vi "Set_Input_file.vi"() -> (2 "输出文件名称":string)   [LabVIEW 2018]
panel:
  in  "版本":string
  in  "输入文件名称：":string
  in  "停止":bool
  in  "确定":bool
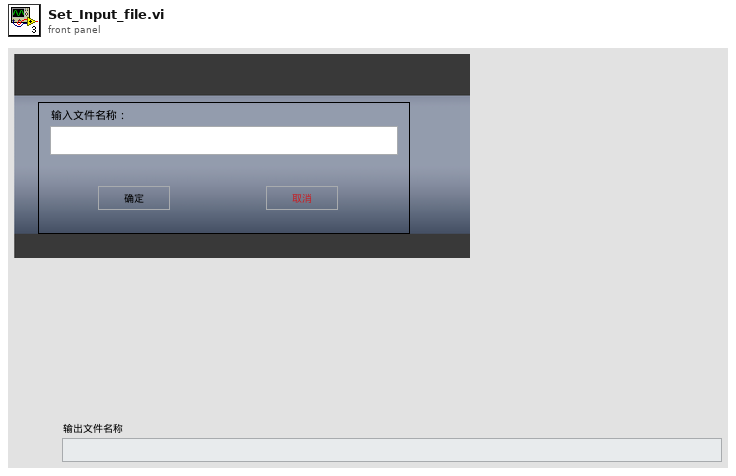
[diagram p1: front panel]
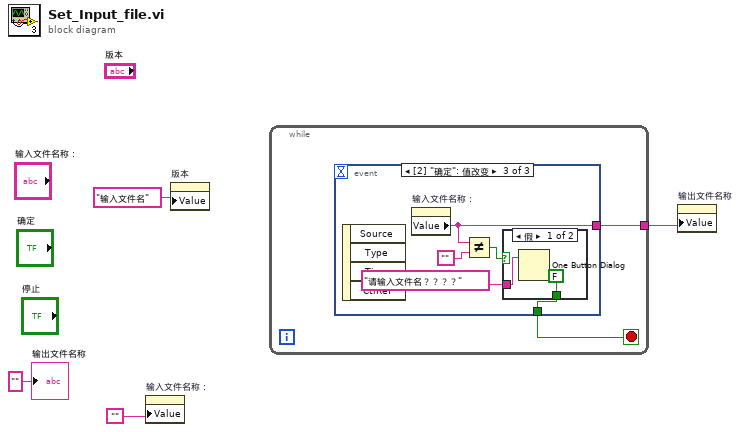
[diagram p0: block diagram]
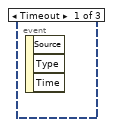
[diagram p2: hidden frame]
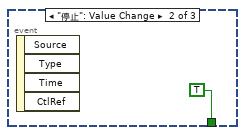
[diagram p3: hidden frame]
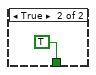
[diagram p4: hidden frame]
diagram:
  n1 = property on="输入文件名称：" class="Str"("Value"="") -> ()  [unwired: 2 in, 2 out]
  n2 = property on="版本" class="Str"("Value"="输入文件名" ("版本")) -> ()  [unwired: 2 in, 2 out]
  n3 = while {
    tunnel: [w5] -> w3
    stop <- w6 stop-if-true
    n4 = event shown="[2] \"确定\": 值改变" {
      selector: _ -> [_ _ _]
      dyn-events: _ -> [_ _ _]
      timeout: _ -> [_ _ _]
      tunnel: [_ TRUE w9] -> w6
      tunnel: [_ _ w12] -> w5
      event Timeout {
        n5 = event-data() -> ()  [unwired: 1 in, 3 out]
      }
      event "停止": Value Change {
        n6 = event-data() -> ()  [unwired: 1 in, 4 out]
      }
      event "确定": Value Change {
        n7 = event-data() -> ()  [unwired: 1 in, 4 out]
        n8 = property on="输入文件名称：" class="Str"() -> ("Value"=w12:string)  [unwired: 2 in, 2 out]
        n9 = Not Equal?(x=w12, y="") -> (x != y?=w10:bool)
        n10 = case shown="假" w10 {
          tunnel: [FALSE TRUE] -> w9
          tunnel: "请输入文件名？？？？" -> [w13 _]
          frame False {
            n11 = One Button Dialog(message=w13) -> ()  [unwired: 1 in, 1 out]
          }
          frame True {
          }
        }
      }
    }
  }
  n12 = property on="输出文件名称" class="Str"("Value"=w3) -> ()  [unwired: 2 in, 2 out]
  "输出文件名称" <- "" ("输出文件名称")
